vi "Option to string.vi"(11 "String in":string) -> (3 "String out":string)   [LabVIEW 2015]
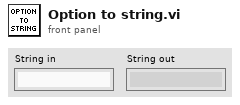
[diagram p1: front panel]
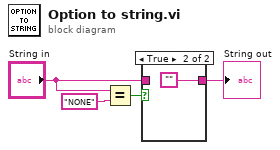
[diagram p0: block diagram]
diagram:
  n1 = Equal?(x="String in", y="NONE") -> (x = y?=w4:bool)
  n2 = case shown="True" w4 {
    tunnel: "String in" -> [w5 _]
    tunnel: [w5 ""] -> w1
    frame False {
    }
    frame True {
    }
  }
  "String out" <- w1
